vi "CompRunInitialization.vi"() -> ()   [LabVIEW 2024]
panel:
  in  "Frequency Channel":enum16{"Channel 1", "Channel 2", "Channel 3"}(ring)
  in  "Cancel":bool
  in  "TempType":T1(ring)=enum."2"
  in  "Step Soak":T2(ring)=enum."5 mins"
  in  "Final Soak":T2(ring)=enum."5 mins"
  in  "Slew Rate":enum16{"0.5", "1", "2"}(ring)=enum."1"
  in  "Initial Soak":T2(ring)=enum."5 mins"
  in  "V inj Min":dbl min=0.0 max=20.0 format="%.4f"
  in  "OK":bool
  in  "Gate Time":T3(ring)=enum."1.0 second"
  in  "Vinj Max":dbl=6.0 min=-6.0 max=20.0 format="%.4f"
  in  "Dmm Readings":i8=5 min=0 max=5 step=1
  in  "Tolerence":dbl=0.01 min=0.001 max=100.0 format="%.2f"
  in  "Nominal":dbl=1.0 min=0.0 max=1000.0 format="%.4f"
  # "Parameters Parameters"
  # "MHz"
  # "PPM"
  # "V"
  # "V"
  # "Temperature"
  # "Frequency Counter"
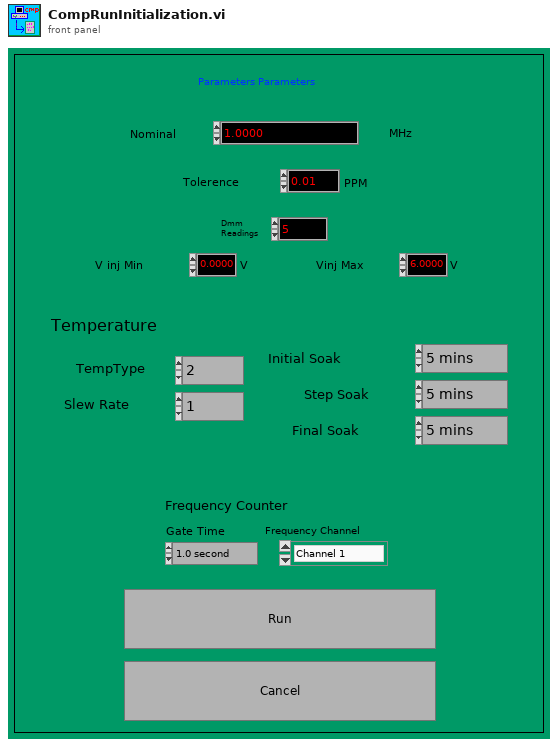
[diagram p1: front panel]
types:
  T1 = enum16{"1", "2", "3", "4", "5", "6", "7", "8", "9", "10", "11", "12", "13", "14", "15"}
  T2 = enum16{"1 min", "5 mins", "10 mins", "20 mins", "30 mins", "40 mins", "50 mins", "1 hour", "2 hours", "3 hours"}
  T3 = enum16{"0.1 second", "1.0 second", "10.0 second"}
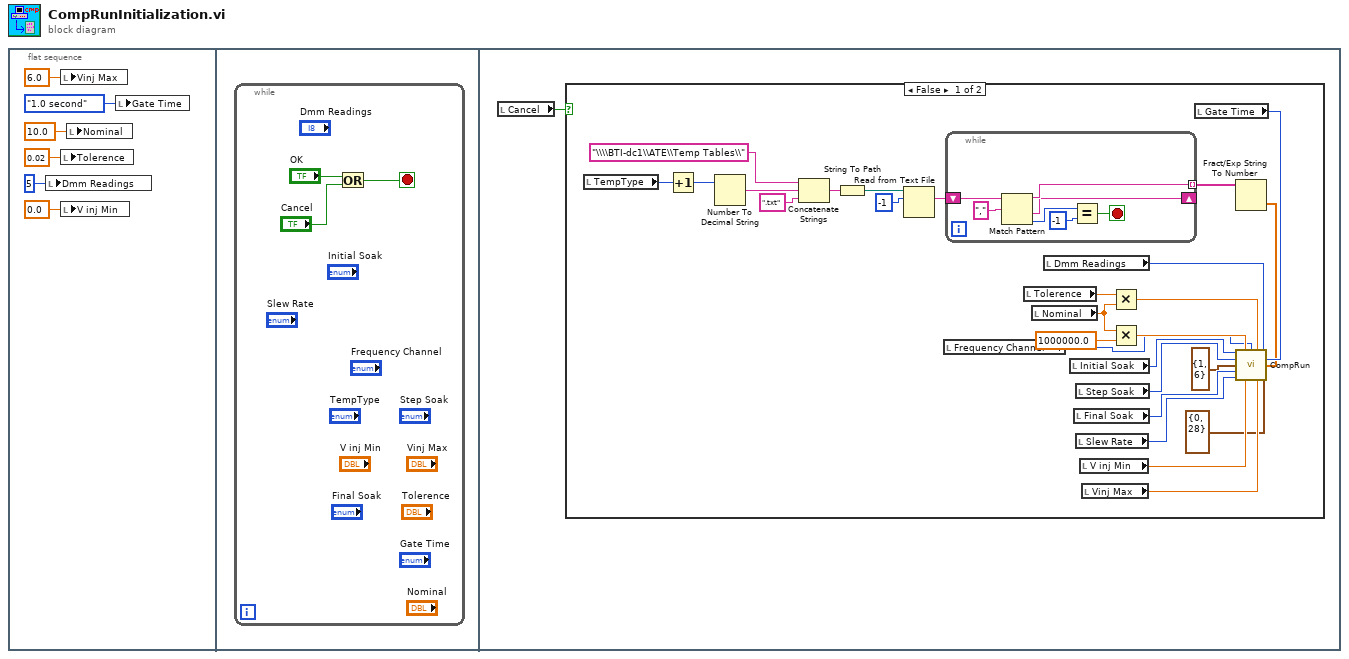
[diagram p0: block diagram]
diagram:
  n1 = flat-sequence {
    frame #0 {
      n2 = local write "Dmm Readings"(i8 5 ("Dmm Readings")) -> ()
      n3 = local write "Vinj Max"(6.0 ("Vinj Max")) -> ()
      n4 = local write "Tolerence"(0.02 ("Tolerence")) -> ()
      n5 = local write "V inj Min"(0.0 ("V inj Min")) -> ()
      n6 = local write "Nominal"(10.0 ("Nominal")) -> ()
      n7 = local write "Gate Time"(T3."1.0 second" ("Gate Time")) -> ()
    }
    frame #1 {
      n8 = while {
        stop <- w9 stop-if-true
        n9 = Or(x="OK", y="Cancel") -> (x .or. y?=w9:bool)
      }
    }
    frame #2 {
      n10 = local read "Cancel"() -> (w10:bool)
      n11 = case shown="False" w10 {
        frame False {
          n12 = local read "TempType"() -> (w26:T1)
          n13 = Increment(x=w26) -> (x+1=w25:T1)
          n14 = Number To Decimal String(number=w25) -> (decimal integer string=w33:string)  [unwired: 1 in]
          n15 = Concatenate Strings("\\\\BTI-dc1\\ATE\\Temp Tables\\" ("search string/char (-)"), w33, ".txt" ("string")) -> (w34:string)
          n16 = String To Path(string=w34) -> (path=w35:path)
          n17 = Read from Text File(file (use dialog)=w35, count=-1) -> (text=w36:string)  [unwired: 2 in, 3 out]
          n18 = local read "Frequency Channel"() -> (w11:enum16{"Channel 1", "Channel 2", "Channel 3"})
          n19 = while {
            tunnel: [w42] -> w37 mode=indexing
            shift-right: [w41] -> _
            shift-left: w36 -> [w40]
            stop <- w43 stop-if-true
            n20 = Match Pattern(string=w40, regular expression="," ("search string/char (-)")) -> (before substring=w42:string, after substring=w41:string, offset past match=w38:i32)  [unwired: 1 in, 1 out]
            n21 = Equal?(x=w38, y=-1) -> (x = y?=w43:bool)
          }
          n22 = local read "Tolerence"() -> (w27:dbl)
          n23 = local read "Nominal"() -> (w28:dbl)
          n24 = local read "Dmm Readings"() -> (w22:i8)
          n25 = local read "Initial Soak"() -> (w20:T2)
          n26 = local read "Final Soak"() -> (w18:T2)
          n27 = local read "Step Soak"() -> (w19:T2)
          n28 = local read "Slew Rate"() -> (w17:enum16{"0.5", "1", "2"})
          n29 = local read "V inj Min"() -> (w15:dbl)
          n30 = local read "Vinj Max"() -> (w16:dbl)
          n31 = Multiply(x=w27, y=w28) -> (x*y=w23:dbl)
          n32 = Multiply(x=w28, y=1000000.0) -> (x*y=w24:dbl)
          n33 = local read "Gate Time"() -> (w21:T3)
          n34 = Fract/Exp String To Number(string=w37) -> (number=w14:dbl[])  [unwired: 3 in, 1 out]
          n35 = call "CompRun.vi"("Initial Soak"=w20, "Nominal"=w24, "Frequency Channel"=w11, "Tolerence"=w23, "Dmm Readings"=w22, "Step Soak"=w19, "Gate Time"=w21, "HP Switcher Address"=cluster{"GPIB":u8, "Address":u8} {"GPIB"=1, "Address"=6}, "Temperature Array"=w14, "Final Soak"=w18, "Slew Rate"=w17, "V inj Min"=w15, "Vinj Max"=w16, "Chamber Address"=cluster{"GPIB #":u8, "Address":u8} {"GPIB #"=0, "Address"=28}) -> ()  [unwired: 2 in]
        }
        frame True {
        }
      }
    }
  }
